vi "BRig_Host__Loop_Producer__tcp_System__v3.vi"(0 "input_strCmd":string, 2 "input_I_SentCmd":bool, 4 "input_hDataQueue":refnum<queue>, 5 "input_error_dataqueue":errorcluster, 6 "input_I_Stop":bool, 8 "input_I_ExpRun":bool) -> (10 "output_I_ExpRun":bool, 12 "output_I_Stop":bool, 16 "output_I_sentCmd":bool, 18 "output_hDataQueue":refnum<queue>, 19 "output_error":errorcluster)   [LabVIEW 2014]
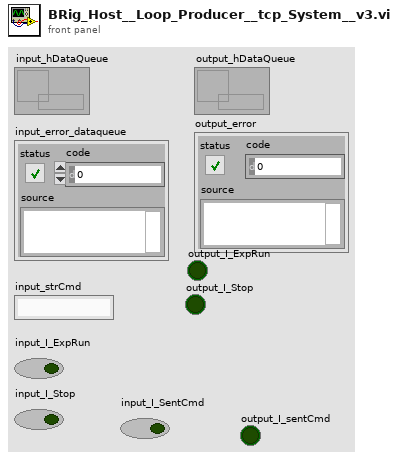
[diagram p1: front panel]
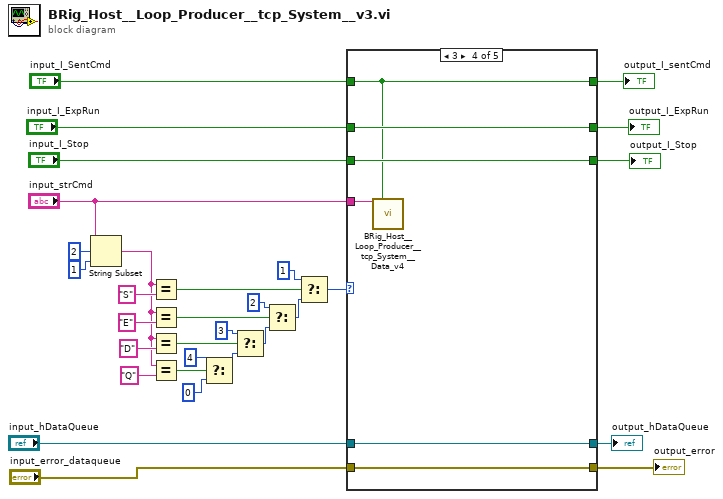
[diagram p0: block diagram]
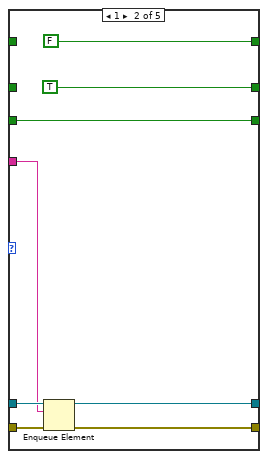
[diagram p3: hidden frame]
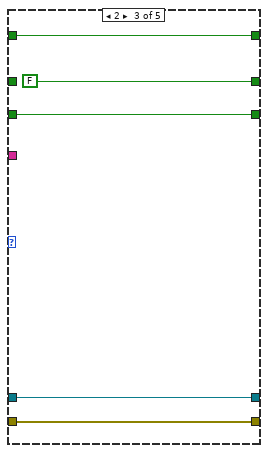
[diagram p4: hidden frame]
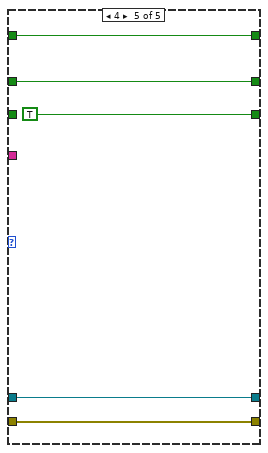
[diagram p5: hidden frame]
diagram:
  n1 = String Subset(string="input_strCmd", offset (0)=2, length (rest)=1 ("offset (0)")) -> (substring=w25:string)
  n2 = Equal?(x=w25, y="S") -> (x = y?=w24:bool)
  n3 = Equal?(x=w25, y="E") -> (x = y?=w23:bool)
  n4 = Equal?(x=w25, y="D") -> (x = y?=w22:bool)
  n5 = Equal?(x=w25, y="Q") -> (x = y?=w21:bool)
  n6 = Select(t=u8 4, s=w21, f=u8 0) -> (s? t:f=w20:u8)
  n7 = Select(t=u8 3, s=w22, f=w20) -> (s? t:f=w19:u8)
  n8 = Select(t=u8 2, s=w23, f=w19) -> (s? t:f=w18:u8)
  n9 = Select(t=u8 1, s=w24, f=w18) -> (s? t:f=w12:u8)
  n10 = case shown="3" w12 {
    tunnel: "input_strCmd" -> [_ w42 _ w51 _]
    tunnel: "input_hDataQueue" -> [w36 w44 w49 w55 w60]
    tunnel: "input_error_dataqueue" -> [w35 w43 w48 w54 w59]
    tunnel: [w36 w41 w49 w55 w60] -> w8
    tunnel: [w35 w40 w48 w54 w59] -> w7
    tunnel: "input_I_ExpRun" -> [w34 _ _ w53 w57]
    tunnel: "input_I_Stop" -> [w33 w39 w47 w52 _]
    tunnel: [w34 TRUE FALSE w53 w57] -> w4
    tunnel: [w33 w39 w47 w52 TRUE] -> w3
    tunnel: "input_I_SentCmd" -> [w32 _ w45 w50 w56]
    tunnel: [w32 FALSE ("f") w45 w50 w56] -> w1
    frame 0, Default {
    }
    frame 1 {
      n11 = Enqueue Element(queue=w44, element=w42, error in (no error)=w43) -> (queue out=w41:refnum<queue>, error out=w40:errorcluster)  [unwired: 1 in, 1 out]
    }
    frame 2 {
    }
    frame 3 {
      n12 = call "BRig_Host__Loop_Producer__tcp_System__Data_v4.vi"("input_strCmd"=w51, "input_I_SentCmd"=w50) -> ()  [unwired: 14 in]
    }
    frame 4 {
    }
  }
  "output_hDataQueue" <- w8
  "output_error" <- w7
  "output_I_ExpRun" <- w4
  "output_I_Stop" <- w3
  "output_I_sentCmd" <- w1
